vi "New Data File.vi"(4 "Plot group":string, 6 "Plot type":T1, 8 "error in (no error)":errorcluster, 9 "New plot if not open":bool, 10 "File":path, 11 "Application Controller in":refnum<class "Application Controller.lvclass">) -> (0 "error out":errorcluster, 3 "Application Controller out":refnum<class "Application Controller.lvclass">)   [LabVIEW 2019, in "Application Controller.lvclass"]
uses:
  Application Controller.lvclass
  Plots/Plot types.ctl
  <vilib>/ActorFramework/Message Enqueuer/Message Enqueuer.lvclass
  Application Controller.lvclass/Application Controller.ctl
  Plots/Plot Messages/Add file Msg/Add file Msg.lvclass/Add file Msg.ctl
  <vilib>/ActorFramework/Message Enqueuer/Message Enqueuer.lvclass/Message Enqueuer.ctl
  <vilib>/ActorFramework/Message Enqueuer/Enqueue.vi
  Plots/Plot Messages/Add file Msg/Add file Msg.lvclass
  C:/Program Files/National Instruments/LabVIEW 2019/vi.lib/ActorFramework/Message/Message.lvclass
  <vilib>/ActorFramework/Message Priority Queue/Priority Enqueue.vi
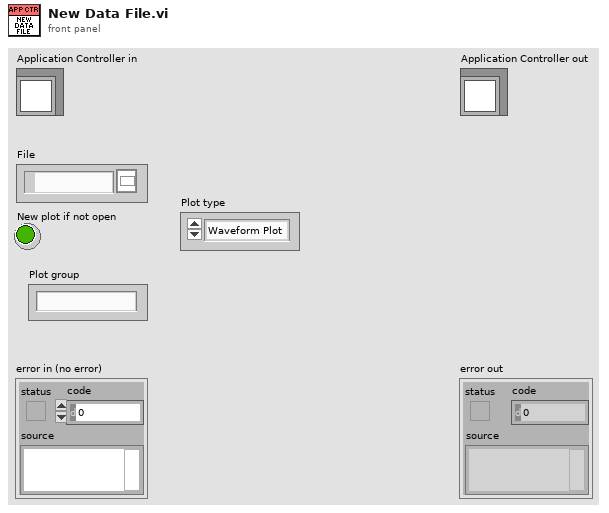
[diagram p1: front panel]
types:
  T1 = typedef "Plot types.ctl" = enum16{"Waveform Plot", "XY Plot", "Full XY"}
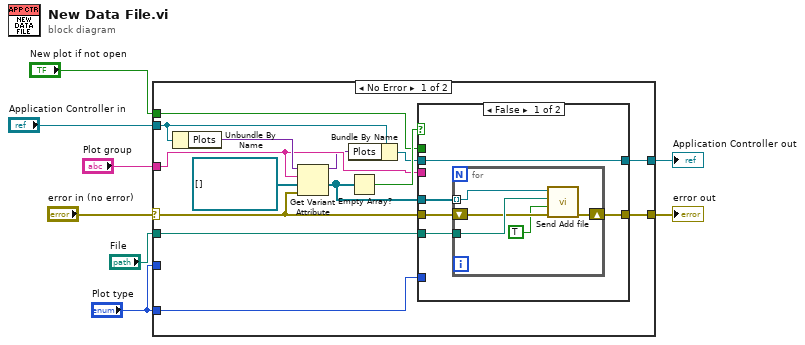
[diagram p0: block diagram]
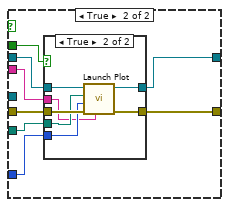
[diagram p2: hidden frame]
diagram:
  n1 = case shown="No Error" "error in (no error)" {
    selector: "error in (no error)" -> [w13 w51]
    tunnel: [w19 w51] -> w4
    tunnel: [w20 w50] -> w3
    tunnel: "Application Controller in" -> [w16 w50]
    tunnel: "File" -> [w21 _]
    tunnel: "New plot if not open" -> [w18 _]
    tunnel: "Plot type" -> [w17 _]
    tunnel: "Plot type" -> [_ _]
    tunnel: "Plot group" -> [w11 _]
    frame No Error {
      n2 = Unbundle By Name(w16) -> ("Plots"=w15:variant)
      n3 = Get Variant Attribute(Variant=w15, name=w11, default value (empty Variant)=refnum<class "Message Enqueuer.lvclass">[] [] ("Pulse plot enqueuers"), error in=w13) -> (duplicate Variant=w9:variant, value=w12:refnum<class "Message Enqueuer.lvclass">[])  [unwired: 2 out]
      n4 = Bundle By Name(cluster=w16, "Plots"=w9) -> (w10:refnum<class "Application Controller.lvclass">)
      n5 = Empty Array?(array=w12) -> (empty?=w22:bool)
      n6 = case shown="False" w22 {
        tunnel: w13 -> [w26 w40]
        tunnel: [w25 w39] -> w19
        tunnel: w10 -> [w24 w38]
        tunnel: [w24 w37] -> w20
        tunnel: w21 -> [w23 w36]
        tunnel: w12 -> [w27 _]
        tunnel: w18 -> [_ w35]
        tunnel: w17 -> [_ w34]
        tunnel: w11 -> [_ w33]
        frame False {
          n7 = for {
            tunnel: w27 -> [w32] mode=indexing
            tunnel: w23 -> [w31]
            shift-right: [w29] -> w25
            shift-left: w26 -> [w30]
            n8 = call "Send Add file.vi"("error in (no error)"=w30, "Insert in front"=TRUE, "File Path Control"=w31, "Message Enqueuer"=w32) -> ("error out"=w29:errorcluster)  [unwired: 6 in, 1 out]
          }
        }
        frame True {
          n9 = case shown="True" w35 {
            tunnel: w40 -> [w42 w49]
            tunnel: [w42 w48] -> w39
            tunnel: w38 -> [w41 w47]
            tunnel: [w41 w46] -> w37
            tunnel: w36 -> [_ w45]
            tunnel: w34 -> [_ w44]
            tunnel: w33 -> [_ w43]
            frame False {
            }
            frame True {
              n10 = call-dynamic "Launch Plot.vi"("Plot group"=w43, "error in (no error)"=w49, "Plot type"=w44, "File Path Control"=w45, "Application Controller in"=w47) -> ("error out"=w48:errorcluster, "Application Controller out"=w46:refnum<class "Application Controller.lvclass">)  [unwired: 4 in, 1 out]
            }
          }
        }
      }
    }
    frame Error {
    }
  }
  "error out" <- w4
  "Application Controller out" <- w3
